vi "Loop Synch.vi"   [LabVIEW 2014]
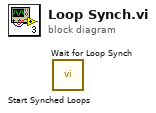
[diagram p0: block diagram]
diagram:
  n1 = call "Start Synched Loops.vi"() -> ()  [unwired: 11 in, 1 out]
  n2 = call "Wait for Loop Synch.vi"() -> ()  [unwired: 11 in, 1 out]
